vi "Floating Intake Immediate.vi"(0 "Setpoint":dbl, 1 "Description":string, 5 "Switch":bool, 7 "Retract":bool, 11 "Command Info In":T1, 12 "Synchronication":enum16{"Start", "Wait"}(ring)) -> (15 "Command Info Out":T1)   [LabVIEW 2018]
doc: "This template is useful for immediate subsystem actions that do not need deadband filtering\n\nBe sure to right-click and select New from Template and save with a new command name."
uses:
  <vilib>/Rock Robotics/WPI/Framework/Command Status Info.ctl
  <vilib>/Rock Robotics/WPI/Framework/Completion Status.ctl
  <vilib>/Rock Robotics/WPI/Framework/Completion Notifier.ctl
  Implementation/Floating Intake Setpoints.ctl
  Implementation/Floating Intake Operations.ctl
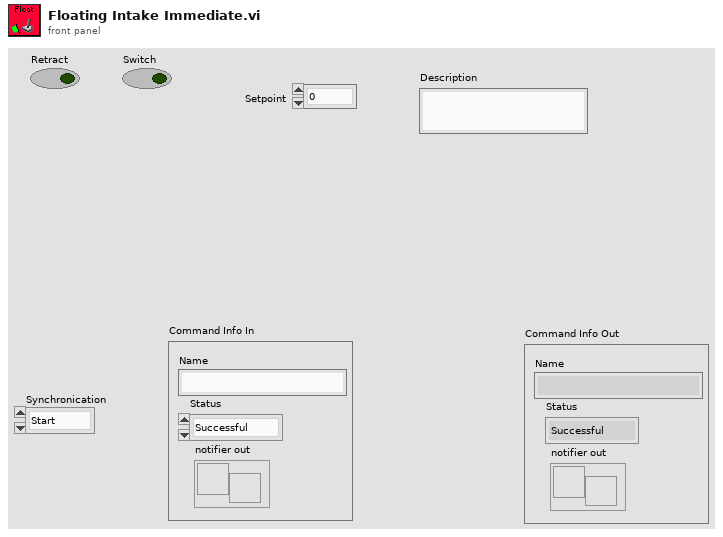
[diagram p1: front panel]
types:
  T1 = typedef "Command Status Info.ctl" = cluster{"Name":string, "Status":T2, "notifier out":T3}
  T2 = typedef "Completion Status.ctl" = enum16{"Successful", "Aborted", "Incomplete"}
  T3 = typedef "Completion Notifier.ctl" = refnum<notifier>
  T4 = typedef "Floating Intake Setpoints.ctl" = cluster{"Operation":T5, "Setpoint":dbl, "Duration":dbl, "Switch":bool, "Retract":bool}
  T5 = typedef "Floating Intake Operations.ctl" = enum16{"Reserve", "Read Current", "Immediate", "Duration"}
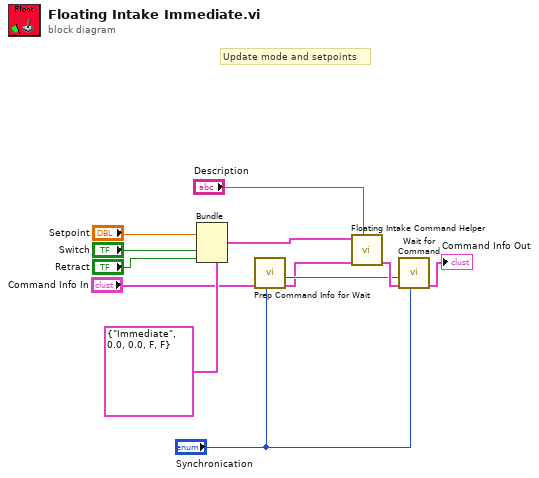
[diagram p0: block diagram]
diagram:
  # "Update mode and setpoints"
  n1 = Bundle(cluster=T4 {"Operation"=enum."Immediate", "Setpoint"=0.0, "Duration"=0.0, "Switch"=FALSE, "Retract"=FALSE} ("SubSystem Data"), "Setpoint"="Setpoint", "Switch"="Switch", "Retract"="Retract") -> (w9:T4)  [unwired: 2 in]
  n2 = call <vilib>:"Prep Command Info for Wait.vi"("Synchronication"="Synchronication", "Command Info"="Command Info In") -> ("Command Info"=w3:T1, "Allocated"=w4:bool)  [unwired: 8 in]
  n3 = call "Floating Intake Command Helper.vi"("Description"="Description", "Command Info In"=w3, "SubSystem Data"=w9) -> ("Command Info Out"=w6:T1)  [unwired: 6 in, 2 out]
  n4 = call <vilib>:"Wait for Command.vi"("Synchronication"="Synchronication", "Command Info in"=w6, "Allocated"=w4) -> ("Command Info out"=→"Command Info Out":T1)  [unwired: 8 in]
